vi "Autoscale Font Size Write 10.vi"(4 "error in (no error)":errorcluster, 5 "Value":bool=TRUE, 6 "Container State":T2, 7 "Display State In":T1={"Autoscale Font Size?"=TRUE, "Alignment"={"horizontal"=enum."left", "vertical"=enum."top"}, "Font"={"Font Name:"="Segoe UI", "Size"=18, "Strikeout?"=FALSE, "Italic?"=FALSE, "Underline?"=FALSE, "Outline?"=FALSE, "Shadow?"=FALSE, "Bold?"=FALSE}, "Text Color"=0, "BG Color"=16777216}) -> (0 "error out":errorcluster, 3 "Display State Out":T1={"Autoscale Font Size?"=TRUE, "Alignment"={"horizontal"=enum."left", "vertical"=enum."top"}, "Font"={"Font Name:"="Segoe UI", "Size"=18, "Strikeout?"=FALSE, "Italic?"=FALSE, "Underline?"=FALSE, "Outline?"=FALSE, "Shadow?"=FALSE, "Bold?"=FALSE}, "Text Color"=0, "BG Color"=16777216})   [LabVIEW 2012, in "String XControl.xctl"]
uses:
  String XControl.xctl
  <vilib>/_xctls/Container State.ctl
  State.ctl
  <vilib>/_xctls/XControlSupport.lvlib
panel:
  # "Replace the Value Control below with a Control of desired type.\nDo not remove this Control or the others from the connector pane.\nDo not change the connector pane pattern.\nThe Value control should always be the third terminal from top on the input side in the connector pane."
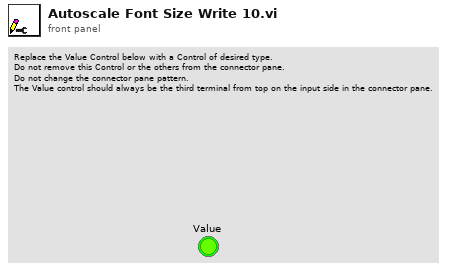
[diagram p1: front panel]
types:
  T1 = typedef "String XControl.xctl/State.ctl" = cluster{"Autoscale Font Size?":bool, "Alignment":cluster{"horizontal":enum16{"left", "center", "right"}, "vertical":enum16{"top", "center", "bottom"}}, "Font":cluster{"Font Name:":string, "Size":i16, "Strikeout?":bool, "Italic?":bool, "Underline?":bool, "Outline?":bool, "Shadow?":bool, "Bold?":bool}, "Text Color":u32, "BG Color":u32}
  T2 = typedef "XControlSupport.lvlib/Container State.ctl" = cluster{"Indicator?":bool, "Run Mode?":bool, " Refnum":refnum<vi>}
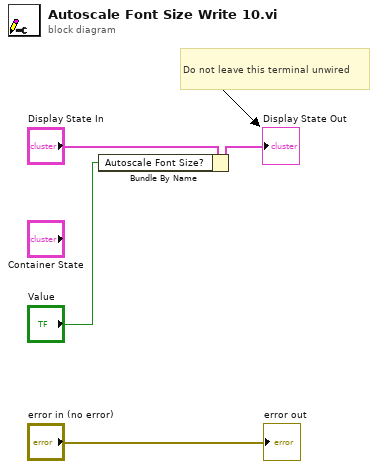
[diagram p0: block diagram]
diagram:
  # "Do not leave this terminal unwired"
  n1 = Bundle By Name(cluster="Display State In", "Autoscale Font Size?"="Value") -> (→"Display State Out":T1)
  "error out" <- "error in (no error)"
